vi "Sigma0.vi"(10 "Value":u32) -> (2 "Sigma 0":u32)   [LabVIEW 2018, in "Crypto.lvlib" / "SHA-256.lvclass"]
uses:
  SHA-256.lvclass
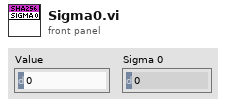
[diagram p1: front panel]
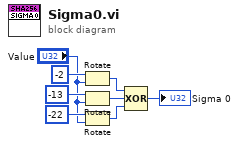
[diagram p0: block diagram]
diagram:
  n1 = Rotate(1:"Value", 2:i16 -2 ("y")) -> (0:w3:u32)
  n2 = Rotate(1:"Value", 2:i16 -13 ("y")) -> (0:w4:u32)
  n3 = Rotate(1:"Value", 2:i16 -22 ("y")) -> (0:w2:u32)
  n4 = Compound Arithmetic op=XOR(w3, w4, w2) -> (→"Sigma 0":u32)
